vi "Player Info.vi"(11 "Hail in":refnum<class "Hail.lvclass">) -> (0 "Defeat Speech":string, 1 "Victory Speech":string, 2 "Name":string, 3 "Hail out":refnum<class "Hail.lvclass">)   [LabVIEW 2015, in "Hail.lvclass"]
uses:
  Hail.lvclass
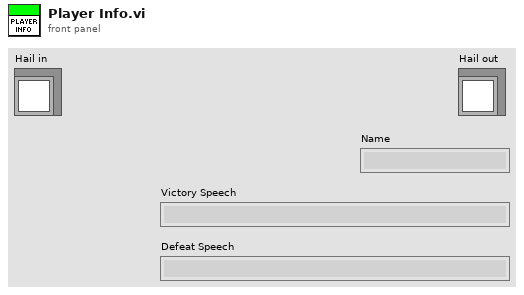
[diagram p1: front panel]
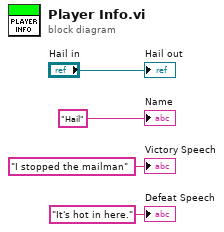
[diagram p0: block diagram]
diagram:
  "Hail out" <- "Hail in"
  "Name" <- "Hail" ("Name")
  "Victory Speech" <- "I stopped the mailman" ("Victory Speech")
  "Defeat Speech" <- "It's hot in here." ("Defeat Speech")
